vi "PH_BeamlineController.ProcEvents.vi"(0 "i ref in":refnum<vi>, 5 "error in (no error)":errorcluster) -> (14 "i ref out":refnum<vi>, 19 "error out":errorcluster)   [LabVIEW 2014, in "PH_BeamlineController.lvlib"]
doc: "This method is used to define the events the object will listen to. Add your own events here."
uses:
  PH_BeamlineController.lvlib
  CS_Core/BaseProcess/BaseProcess.event definition.ctl
  CS_Core/CAEObj/CAEObj.event definition.ctl
  CS_Core/BaseProcess/BaseProcess.descriptor string definition.ctl
  CS_Core/BaseProcess/BaseProcess.lvlib
  PH_Basics/PH_Common/PH_Common.lvlib
  CS_Core/CAEObj/CAEObj.lvlib
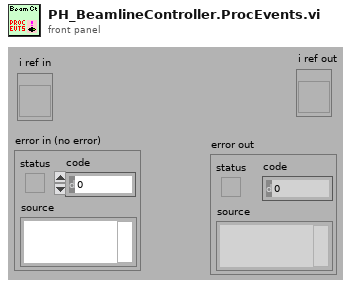
[diagram p1: front panel]
types:
  T1 = typedef "BaseProcess.lvlib/BaseProcess.event definition.ctl" = cluster{"CAEEvtDef":T2, "Data Descriptor":T3}
  T2 = typedef "CAEObj.lvlib/CAEObj.event definition.ctl" = cluster{"URL":string, "enable":bool, "ignoreResID":bool}
  T3 = typedef "BaseProcess.lvlib/BaseProcess.descriptor string definition.ctl" = string
  T4 = typedef "PH_BeamlineController.lvlib/PH_BeamlineController.i attribute.ctl" = cluster{"Vacuum Exp LB":cluster{"Channel":string, "Limit [mbar]":dbl, "Pressure [mbar]":dbl, "GUI Ref":refnum<vi>}, "Sources":T5[], "PA DP Targets":T7[], "Path":cluster{"Source":T6, "PA DP Target":T8, "Target":T9}, "Targets":cluster{"Name":T9, "GUI Ref":refnum<vi>, "Current State":bool, "Wanted State":bool, "Enabled":bool}[], "Status Tags":cluster{"Name":string, "Status":T10}[], "special GUI Refs":T11}
  T5 = typedef "PH_BeamlineController.lvlib/PH_BeamlineController.Source Attributes.ctl" = cluster{"Name":T6, "GUI Ref":refnum<vi>, "Current State":bool, "Wanted State":bool}
  T6 = typedef "PH_BeamlineController.lvlib/PH_BeamlineController.Sources.ctl" = enum16{"None", "YLF", "fs-Frontend", "ns-Frontend", "YLF and ns-Frontend", "fs- and ns-Frontend"}
  T7 = typedef "PH_BeamlineController.lvlib/PH_BeamlineController.PA DP Target Attributes.ctl" = cluster{"Name":T8, "GUI Ref":refnum<vi>, "Current State":bool, "Wanted State":bool, "Enabled":bool}
  T8 = typedef "PH_BeamlineController.lvlib/PH_BeamlineController.PA DP Targets.ctl" = enum16{"None", "Dump PA Delayed Beam", "Dump PA Undelayed Beam", "Dumps PA Delayed and Undelayed Beam"}
  T9 = typedef "PH_BeamlineController.lvlib/PH_BeamlineController.Targets.ctl" = enum16{"None", "PreAmp", "Dump Exp Laserlab", "Exp Laserlab", "Calorimeter", "Dump Exp Laserbay", "Exp Laserbay", "Dump Exp Z6", "Exp Z6"}
  T10 = typedef "PH_StatusHandler.lvlib/PH_StatusHandler.Status.ctl" = i16
  T11 = typedef "PH_BeamlineController.lvlib/PH_BeamlineController.special GUI Refs.ctl" = cluster{"PA-Backreflection-Meas":refnum<vi>, "fs_Synchrolock_Watch":refnum<vi>}
  T12 = typedef "PH_Common.lvlib/PH_DIM.Event Declarer.ctl" = cluster{"Service Name":string, "Selector":string}
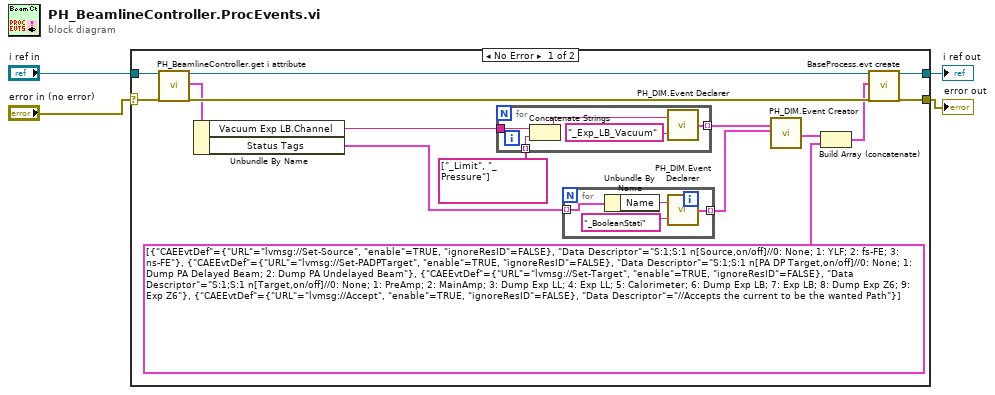
[diagram p0: block diagram]
diagram:
  n1 = case shown="No Error" "error in (no error)" {
    selector: "error in (no error)" -> [w14 w29]
    tunnel: "i ref in" -> [w17 w30]
    tunnel: [w16 w30] -> w3
    tunnel: [w15 w29] -> w2
    frame No Error {
      n2 = call "PH_BeamlineController.get i attribute.vi"("i ref in"=w17, "error in (no error)"=w14) -> ("i ref out"=w19:refnum<vi>, "i attribute"=w13:T4, "error out"=w18:errorcluster)  [unwired: 15 in]
      n3 = Unbundle By Name(w13) -> ("Vacuum Exp LB.Channel"=w11:string, "Status Tags"=w7:cluster{"Name":string, "Status":T10}[])
      n4 = for {
        tunnel: [w27] -> w5 mode=indexing
        tunnel: w11 -> [w24]
        tunnel: string[] ["_Limit", "_Pressure"] -> [w25] mode=indexing
        n5 = Concatenate Strings(w24, w25) -> (w26:string)
        n6 = call "PH_DIM.Event Declarer.vi"("Selector"="_Exp_LB_Vacuum" ("URL"), "Service Name"=w26) -> ("declared DIM Event"=w27:T12)
      }
      n7 = for {
        tunnel: [w22] -> w6 mode=indexing
        tunnel: w7 -> [w21] mode=indexing
        n8 = Unbundle By Name(w21) -> ("Name"=w20:string)
        n9 = call "PH_DIM.Event Declarer.vi"("Selector"="_BooleanStati", "Service Name"=w20) -> ("declared DIM Event"=w22:T12)
      }
      n10 = call "PH_DIM.Event Creator.vi"("Trendmessage Services"=w5, "Status Services"=w6) -> ("DIM Service Events"=w12:T1[])  [unwired: 17 in]
      n11 = Build Array (concatenate)(w12, T1[] [{"CAEEvtDef"={"URL"="lvmsg://Set-Source", "enable"=TRUE, "ignoreResID"=FALSE}, "Data Descriptor"="S:1;S:1 n[Source,on/off]//0: None; 1: YLF; 2: fs-FE; 3: ns-FE"}, {"CAEEvtDef"={"URL"="lvmsg://Set-PADPTarget", "enable"=TRUE, "ignoreResID"=FALSE}, "Data Descriptor"="S:1;S:1 n[PA DP Target,on/off]//0: None; 1: Dump PA Delayed Beam; 2: Dump PA Undelayed Beam"}, {"CAEEvtDef"={"URL"="lvmsg://Set-Target", "enable"=TRUE, "ignoreResID"=FALSE}, "Data Descriptor"="S:1;S:1 n[Target,on/off]//0: None; 1: PreAmp; 2: MainAmp; 3: Dump Exp LL; 4: Exp LL; 5: Calorimeter; 6: Dump Exp LB; 7: Exp LB; 8: Dump Exp Z6; 9: Exp Z6"}, {"CAEEvtDef"={"URL"="lvmsg://Accept", "enable"=TRUE, "ignoreResID"=FALSE}, "Data Descriptor"="//Accepts the current to be the wanted Path"}] ("array")) -> (w9:T1[])
      n12 = call "BaseProcess.evt create.vi"("i ref in"=w19, "newEvents"=w9, "error in (no error)"=w18) -> ("i ref out"=w16:refnum<vi>, "error out"=w15:errorcluster)  [unwired: 13 in, 2 out]
    }
    frame Error {
    }
  }
  "i ref out" <- w3
  "error out" <- w2
